vi "SVI_Calculate_checksum.vi"(1 "Message":string, 2 "Type":enum16{"ReadableChars", "SpellmanMPS"}(ring)) -> (0 "Calculated checksum":string)   [LabVIEW 2014]
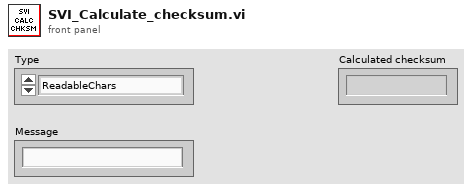
[diagram p1: front panel]
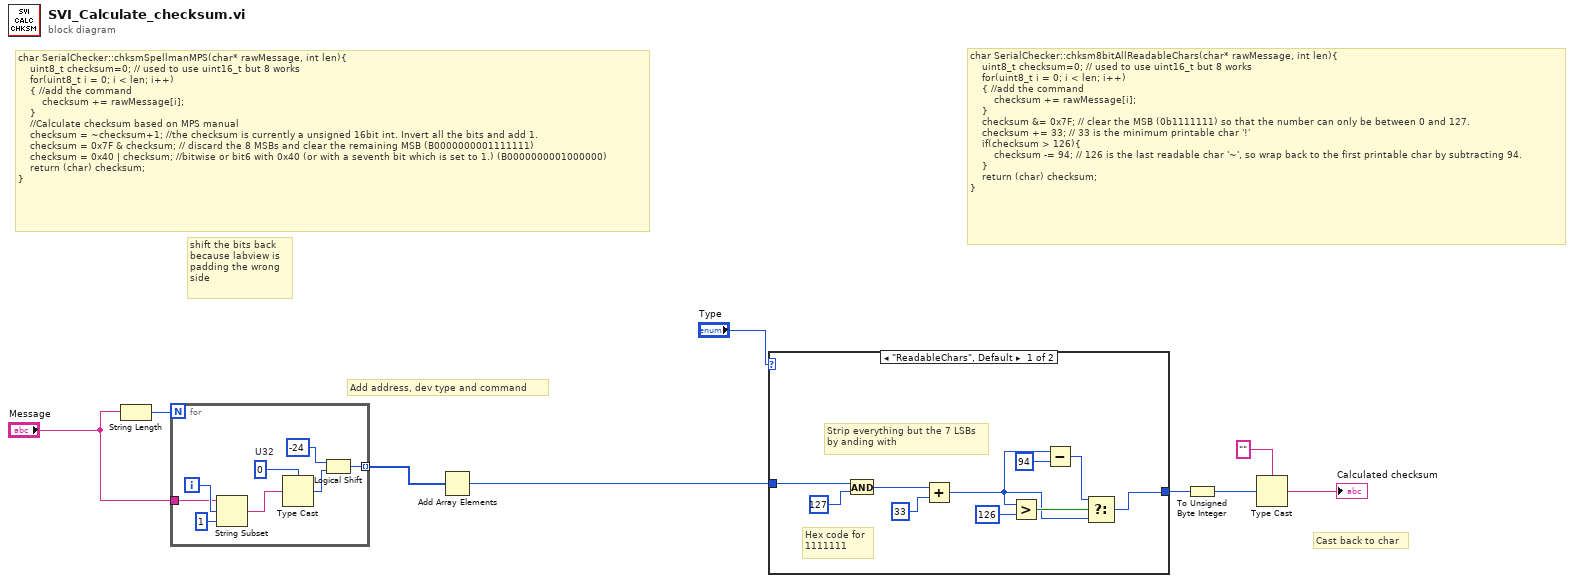
[diagram p0: block diagram]
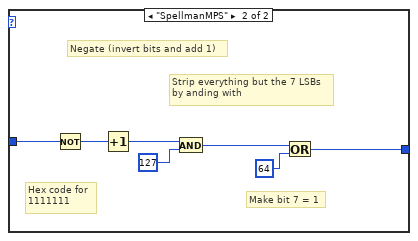
[diagram p2: hidden frame]
diagram:
  # "Cast back to char"
  # "char SerialChecker::chksmSpellmanMPS(char* rawMessage, int len){\n    uint8_t checksum=0; // used to use uint16_t but 8 works\n    for(uint8_t i = 0; i < len; i++)\n    { //add the command\n        checksum += rawMessage[i];\n    }\n    //Calculate checksum based on MPS manual\n    checksum = ~checksum+1; //the checksum is currently a unsigned 16bit int. Invert all the bits and add 1.\n    checksum = 0x7F & checksum; // discard the 8 MSBs and clear the remaining MSB (B0000000001111111)\n    checksum = 0x40 | checksum; //bitwise or bit6 with 0x40 (or with a seventh bit which is set to 1.) (B0000000001000000)\n    return (char) checksum;\n}"
  # "char SerialChecker::chksm8bitAllReadableChars(char* rawMessage, int len){\n    uint8_t checksum=0; // used to use uint16_t but 8 works\n    for(uint8_t i = 0; i < len; i++)\n    { //add the command\n        checksum += rawMessage[i];\n    }\n    checksum &= 0x7F; // clear the MSB (0b1111111) so that the number can only be between 0 and 127.\n    checksum += 33; // 33 is the minimum printable char '!'\n    if(checksum > 126){\n        checksum -= 94; // 126 is the last readable char '~', so wrap back to the first printable char by subtracting 94.\n    }\n    return (char) checksum;\n}"
  # "shift the bits back\nbecause labview is \npadding the wrong\nside"
  # "Add address, dev type and command"
  n1 = String Length(string="Message") -> (length=w8:i32)
  n2 = for {
    N: w8 -> [_]
    tunnel: "Message" -> [w16]
    tunnel: [w10] -> w7 mode=indexing
    i -> [w17]
    w15 = u32 0  # U32
    n3 = String Subset(string=w16, offset (0)=w17, length (rest)=1 ("length (rest)")) -> (substring=w14:string)
    n4 = Type Cast(type=w15, x=w14) -> (*(type *) &x=w12:u32)
    n5 = Logical Shift(y=i16 -24, x=w12) -> (x << y=w10:u32)
  }
  n6 = Add Array Elements(numeric array=w7) -> (sum=w1:u32)
  n7 = case shown="\"ReadableChars\", Default" "Type" {
    tunnel: w1 -> [w19 w29]
    tunnel: [w24 w33] -> w3
    frame "ReadableChars", Default {
      # "Hex code for\n1111111"
      # "Strip everything but the 7 LSBs\nby anding with"
      n8 = And(x=w19, y=u32 127) -> (x .and. y?=w18:u32)
      n9 = Add(x=w18, y=u32 33) -> (x+y=w21:u32)
      n10 = Greater?(x=w21, y=u32 126) -> (0:w25:bool)
      n11 = Subtract(x=w21, y=u32 94) -> (x-y=w22:u32)
      n12 = Select(t=w22, s=w25, f=w21) -> (s? t:f=w24:u32)
    }
    frame "SpellmanMPS" {
      # "Hex code for\n1111111"
      # "Strip everything but the 7 LSBs\nby anding with"
      # "Negate (invert bits and add 1)"
      # "Make bit 7 = 1"
      n13 = Not(x=w29) -> (.not. x?=w31:u32)
      n14 = Increment(x=w31) -> (x+1=w30:u32)
      n15 = And(x=w30, y=u32 127) -> (x .and. y?=w28:u32)
      n16 = Or(x=w28, y=u32 64) -> (x .or. y?=w33:u32)
    }
  }
  n17 = To Unsigned Byte Integer(number=w3) -> (unsigned 8bit integer=w6:u8)
  n18 = Type Cast(type="", x=w6) -> (*(type *) &x=→"Calculated checksum":string)
